vi "Update Data.vi"(9 "queue out":refnum<queue>, 10 "data":variant, 11 "cluster in":T1) -> (1 "data element  2":dbl, 2 "data element  1":dbl, 3 "cluster out":T1)   [LabVIEW 2016]
doc: "update sensor data and data chunk data, and if necessary recording data as well."
uses:
  DataLoopCluster.ctl
  SignalType.ctl
  range_cluster.ctl
  DataType.ctl
  data_command_enum.ctl
  sensor_data.ctl
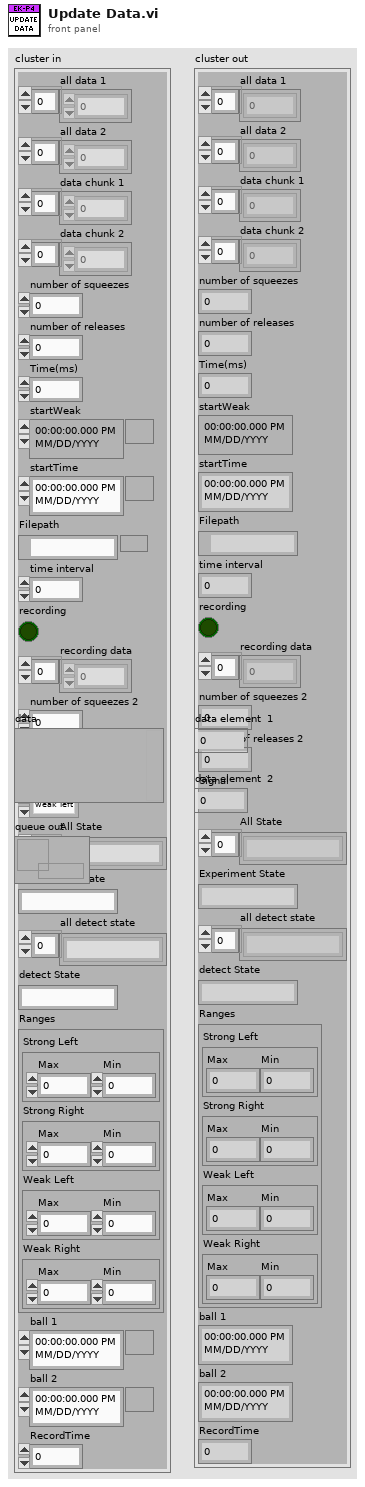
[diagram p1: front panel]
types:
  T1 = typedef "DataLoopCluster.ctl" = cluster{"all data 1":dbl[], "all data 2":dbl[], "data chunk 1":dbl[], "data chunk 2":dbl[], "number of squeezes":u16, "number of releases":u16, "Time(ms)":i64, "startWeak":timestamp, "startTime":timestamp, "Filepath":path, "time interval":u16, "recording":bool, "recording data":dbl[], "number of squeezes 2":u16, "number of releases 2":u16, "Signal":T2, "All State":string[], "Experiment State":string, "all detect state":string[], "detect State":string, "Ranges":cluster{"Strong Left":T3, "Strong Right":T3, "Weak Left":T3, "Weak Right":T3}, "ball 1":timestamp, "ball 2":timestamp, "RecordTime":u16}
  T2 = typedef "SignalType.ctl" = enum16{"weak left", "weak right", "strong left", "strong right"}
  T3 = typedef "range_cluster.ctl" = cluster{"Max":dbl, "Min":dbl}
  T4 = typedef "sensor_data.ctl" = cluster{"Data":dbl[], "Data 2":dbl[]}
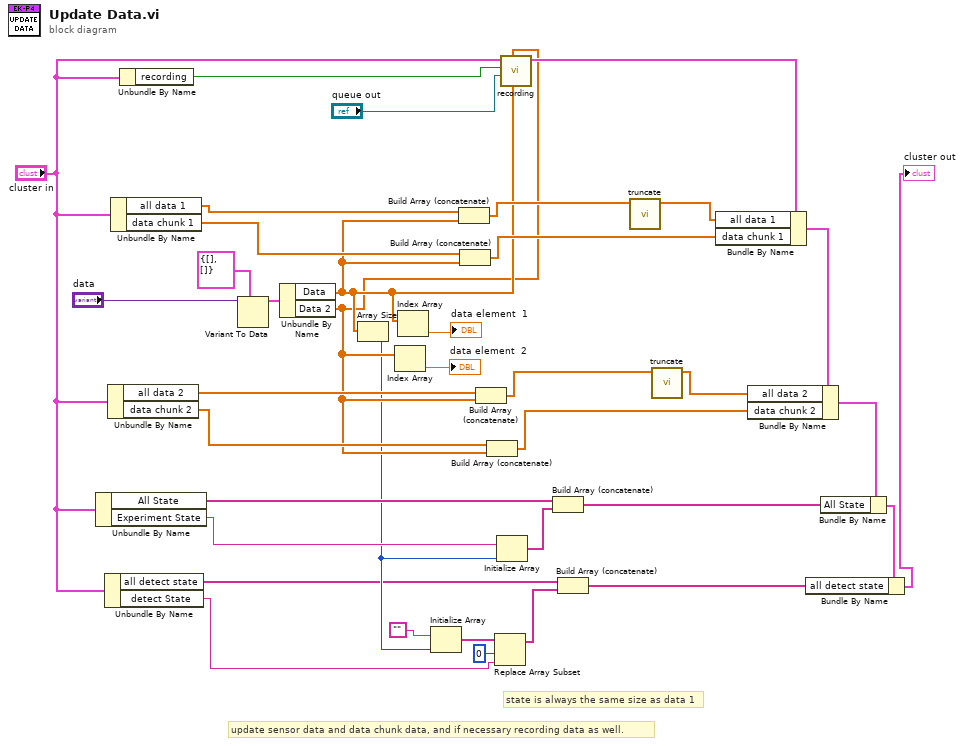
[diagram p0: block diagram]
diagram:
  # "state is always the same size as data 1"
  # "update sensor data and data chunk data, and if necessary recording data as well."
  n1 = Unbundle By Name("cluster in") -> ("All State"=w19:string[], "Experiment State"=w18:string)
  n2 = Unbundle By Name("cluster in") -> ("all detect state"=w9:string[], "detect State"=w2:string)
  n3 = Unbundle By Name("cluster in") -> ("all data 2"=w35:dbl[], "data chunk 2"=w36:dbl[])
  n4 = Unbundle By Name("cluster in") -> ("all data 1"=w31:dbl[], "data chunk 1"=w29:dbl[])
  n5 = Unbundle By Name("cluster in") -> ("recording"=w27:bool)
  n6 = Variant To Data(type=T4 {"Data"=[], "Data 2"=[]} ("cluster"), Variant="data") -> (data=w33:T4)  [unwired: 1 in, 1 out]
  n7 = Unbundle By Name(w33) -> ("Data"=w13:dbl[], "Data 2"=w12:dbl[])
  n8 = Array Size(array=w13) -> (size(s)=w10:i32)
  n9 = Index Array(array=w12) -> (element=→"data element  2":dbl)  [unwired: 1 in]
  n10 = Index Array(array=w13) -> (element=→"data element  1":dbl)  [unwired: 1 in]
  n11 = Initialize Array("", w10) -> (w4:string[])
  n12 = Build Array (concatenate)(w31, w13) -> (w23:dbl[])
  n13 = Build Array (concatenate)(w29, w13) -> (w30:dbl[])
  n14 = Build Array (concatenate)(w35, w12) -> (w21:dbl[])
  n15 = Build Array (concatenate)(w36, w12) -> (w37:dbl[])
  n16 = Replace Array Subset(array=w4, new element=w2, index=0) -> (w1:string[])
  n17 = Initialize Array(w18, w10) -> (w16:string[])
  n18 = call "recording.vi"("Data"=w13, "Data 2"=w12, "Queue in"="queue out", "recording"=w27, "cluster in in"="cluster in") -> ("cluster out"=w26:T1)  [unwired: 6 in]
  n19 = Build Array (concatenate)(w19, w16) -> (w14:string[])
  n20 = Build Array (concatenate)(w9, w1) -> (w7:string[])
  n21 = call "truncate.vi"("Array in"=w23) -> ("Array out"=w22:dbl[])  [unwired: 10 in]
  n22 = call "truncate.vi"("Array in"=w21) -> ("Array out"=w20:dbl[])  [unwired: 10 in]
  n23 = Bundle By Name(cluster=w26, "all data 1"=w22, "data chunk 1"=w30) -> (w34:T1)
  n24 = Bundle By Name(cluster=w34, "all data 2"=w20, "data chunk 2"=w37) -> (w15:T1)
  n25 = Bundle By Name(cluster=w15, "All State"=w14) -> (w8:T1)
  n26 = Bundle By Name(cluster=w8, "all detect state"=w7) -> (→"cluster out":T1)
